vi "Find IntelliSense Control [obj].vi"(0 "IntelliSenseStringControl":refnum<class "IntelliSenseStringControl.lvclass">) -> (1 "Found IntelliSenseStringControl":refnum<class "IntelliSenseStringControl.lvclass">, 2 "Other IntelliSense String []":refnum<class "IntelliSenseStringControl.lvclass">[](array[class]), 3 "Found?":bool)   [LabVIEW 2016, in "StringIntelliSense.lvlib" / "IntelliSenseStringControl.lvclass"]
uses:
  IntelliSenseStringControl.lvclass
  IntelliSenseStringControl.lvclass/IntelliSenseStringControl.ctl
  StringMonitorUserData.vi
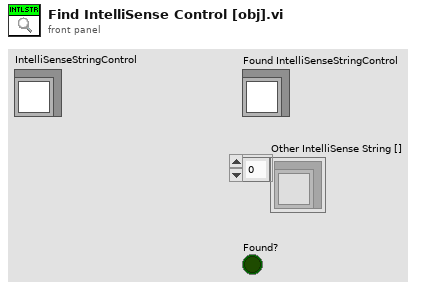
[diagram p1: front panel]
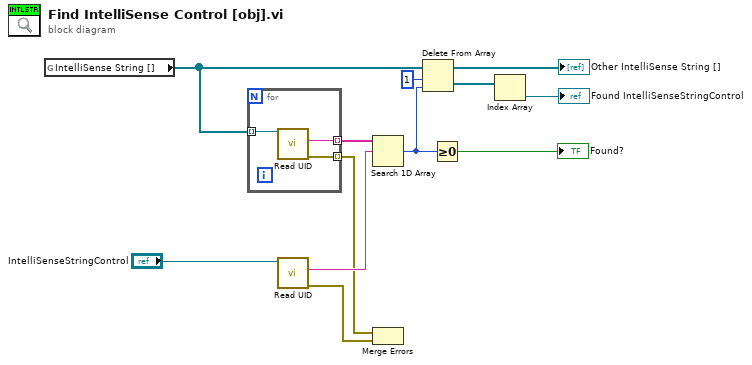
[diagram p0: block diagram]
diagram:
  n1 = global read "StringMonitorUserData.vi" "IntelliSense String []"() -> (w1:refnum<class "IntelliSenseStringControl.lvclass">[])
  n2 = for {
    tunnel: w1 -> [w15] mode=indexing
    tunnel: [w14] -> w12 mode=indexing
    tunnel: [w13] -> w6 mode=indexing
    n3 = call "Read UID.vi"("IntelliSenseStringControl in"=w15) -> ("error out"=w13:errorcluster, "UID"=w14:string)  [unwired: 8 in, 1 out]
  }
  n4 = call "Read UID.vi"("IntelliSenseStringControl in"="IntelliSenseStringControl") -> ("error out"=w5:errorcluster, "UID"=w11:string)  [unwired: 8 in, 1 out]
  n5 = Search 1D Array(1D array=w12, element=w11) -> (index of element=w8:i32)  [unwired: 1 in]
  n6 = Merge Errors(w6, w5) -> ()  [unwired: 1 out]
  n7 = Delete From Array(array=w1, length=1, index=w8) -> (deleted portion=w9:refnum<class "IntelliSenseStringControl.lvclass">[], array with subset deleted=→"Other IntelliSense String []":refnum<class "IntelliSenseStringControl.lvclass">[])
  n8 = Greater Or Equal To 0?(x=w8) -> (x >= 0?=→"Found?":bool)
  n9 = Index Array(array=w9) -> (element=→"Found IntelliSenseStringControl":refnum<class "IntelliSenseStringControl.lvclass">)  [unwired: 1 in]
